vi "sub_bool.vi"() -> ()   [LabVIEW 2019]
uses:
  <vilib>/RTI DDS Toolkit/Types/RTI DDS Advanced Writer Configuration.ctl
  <vilib>/RTI DDS Toolkit/VIs/AdvancedCreateWriter_Bool.vi
  <vilib>/RTI DDS Toolkit/VIs/Read_Bool.vi
  <vilib>/RTI DDS Toolkit/Library/LVDDS_library.lvlib
panel:
  out "error out":errorcluster
  in  "Topic Name":string="rt/subbool"
  in  "stop":bool
  out "Data":bool
  in  "dt":u32=500
  in  "Advanced Writer Configuration":T1={"typeName"="std_msgs::msg::dds_::Bool_", "keyName"="", "domainParticipantQoSProfile"="", "dataWriterQoSProfile"="", "forceArrayMapping?"=FALSE, "forceUnboundedString?"=FALSE}
  in  "Domain Id":u32
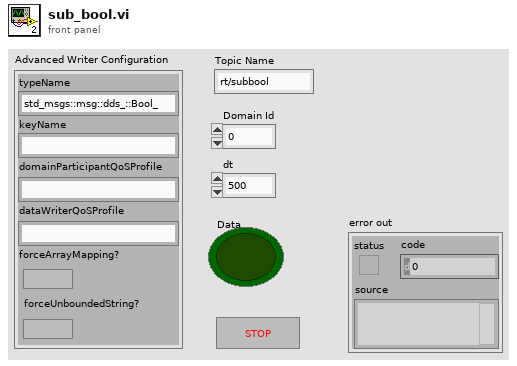
[diagram p1: front panel]
types:
  T1 = typedef "LVDDS_library.lvlib/RTI DDS Advanced Writer Configuration.ctl" = cluster{"typeName":string, "keyName":string, "domainParticipantQoSProfile":string, "dataWriterQoSProfile":string, "forceArrayMapping?":bool, "forceUnboundedString?":bool}
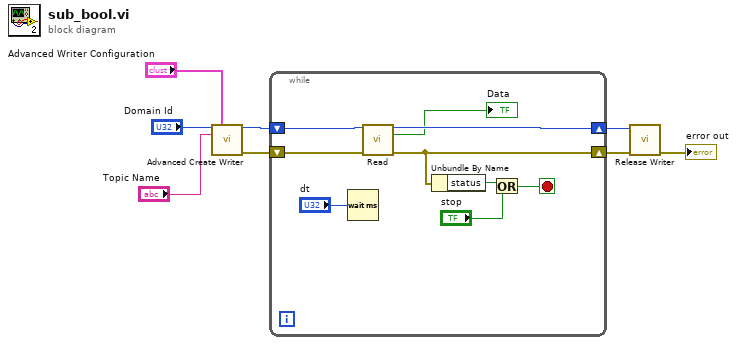
[diagram p0: block diagram]
diagram:
  n1 = call-poly <vilib>:"Advanced Create Writer.vi"("Domain Id"="Domain Id", "Advanced Writer Configuration"="Advanced Writer Configuration", "Topic Name"="Topic Name") -> ("DDS Object Ref"=w8:u64, "error out"=w5:errorcluster)  [unwired: 11 in]
  n2 = while {
    shift-right: [w16] -> w7
    shift-left: w8 -> [w17]
    shift-right: [w14] -> w6
    shift-left: w5 -> [w15]
    stop <- w12 stop-if-true
    n3 = Wait (ms)(milliseconds to wait="dt") -> ()  [unwired: 1 out]
    n4 = call-poly <vilib>:"Read.vi"("DDS Object Ref in"=w17, "error in (no error)"=w15) -> ("DDS Object Ref out"=w16:u64, "Data"=→"Data":bool, "error out"=w14:errorcluster)  [unwired: 9 in, 2 out]
    n5 = Unbundle By Name(w14) -> ("status"=w13:bool)
    n6 = Or(x=w13, y="stop") -> (x .or. y?=w12:bool)
  }
  n7 = call <vilib>:"Release Writer.vi"("error in (no error)"=w6, "DDS Object Ref"=w7) -> ("error out"=→"error out":errorcluster)  [unwired: 9 in]
